vi "Write Start A-Scan Array.vi"(8 "error in (no error)":errorcluster, 10 "Start A-Scan Array":u32[](array[numeric]), 11 "NuFern in":refnum<class "NuFern.lvclass">) -> (0 "error out":errorcluster, 3 "NuFern out":refnum<class "NuFern.lvclass">)   [LabVIEW 2015, in "NuFern.lvclass"]
uses:
  NuFern.lvclass
  NuFern.lvclass/NuFern.ctl
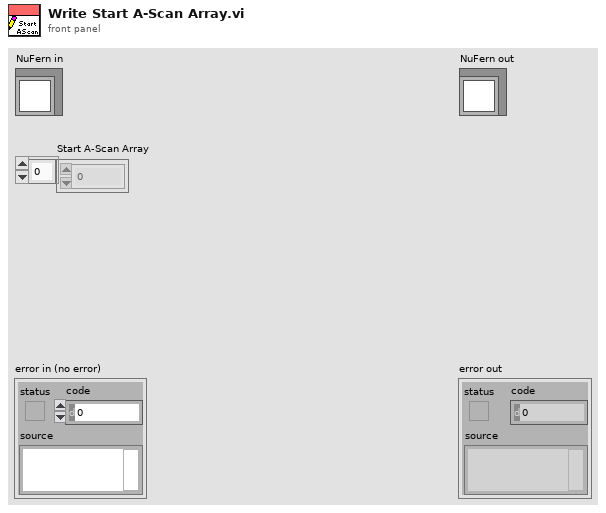
[diagram p1: front panel]
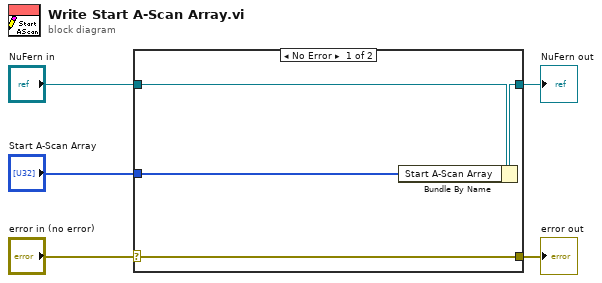
[diagram p0: block diagram]
diagram:
  n1 = case shown="No Error" "error in (no error)" {
    selector: "error in (no error)" -> [w9 w10]
    tunnel: [w9 w10] -> w4
    tunnel: [w7 w11] -> w2
    tunnel: "NuFern in" -> [w8 w11]
    tunnel: "Start A-Scan Array" -> [w6 _]
    frame No Error {
      n2 = Bundle By Name(cluster=w8, "Start A-Scan Array"=w6) -> (w7:refnum<class "NuFern.lvclass">)
    }
    frame Error {
    }
  }
  "error out" <- w4
  "NuFern out" <- w2
